vi "max points enum to number.vi"(11 "Max Sample Points":T1(ring)) -> (3 "Value":i32)   [LabVIEW 2020]
panel:
  in  "Maximum Sample Points (500)":i32(ring)=500 items=["50"=50, "100"=100, "250"=250, "500"=500, "1000"=1000, "2500"=2500, "5K"=5000, "10K"=10000, "25K"=25000, "50K"=50000, "100K"=100000, "250K"=250000, "500K"=500000, "1M"=1000000, "2M"=2000000, "2.5M"=2500000, "5M"=5000000, "10M"=10000000, "25M"=25000000, "50M"=50000000, "100M"=100000000]
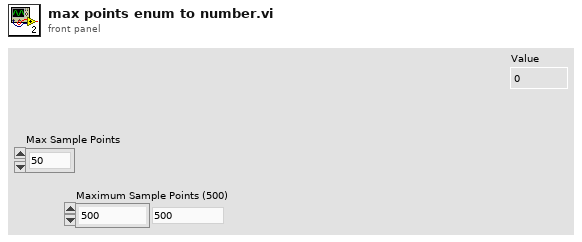
[diagram p1: front panel]
types:
  T1 = enum16{"50", "100", "250", "500", "1000", "2500", "5K", "10K", "25K", "50K", "100K", "250K", "500K", "1M", "2M", "2.5M", "5M", "10M", "25M", "50M", "100M"}
  T2 = typedef "LVStringsAndValuesArrayTypeDef_I32.ctl" = cluster{"String":string, "Value":i32}[]
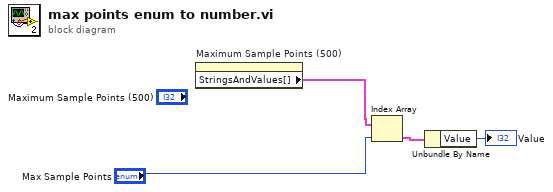
[diagram p0: block diagram]
diagram:
  n1 = property on="Maximum Sample Points (500)" class="Ring (strict)"() -> ("StringsAndValues[]"=w4:T2)  [unwired: 2 in, 2 out]
  n2 = Index Array(array=w4, index="Max Sample Points") -> (element=w2:cluster{"String":string, "Value":i32})
  n3 = Unbundle By Name(w2) -> ("Value"=→"Value":i32)
